vi "Calculate Spot Profile (SubVI).vi"(0 "step":sgl=0.1, 1 "z":sgl, 5 "N points":i32=16, 6 "CUDA/SLM error out":errorcluster, 7 "y":sgl, 8 "CGH out":u8[][](array[numeric]), 9 "x":sgl, 10 "xz-plane":bool) -> (2 "error out":errorcluster, 3 "Spot profile":sgl[][](graph)=[[0.054696757, 0.08603831, 0.118001305, 0.14888857, 0.17700168, 0.20075542, 0.21878594, 0.23004508, 0.2338732, 0.23004507, 0.21878591, 0.20075536, 0.17700155, 0.14888844, 0.118001245, 0.08603819], [0.086038314, 0.13533889, 0.18561684, 0.23420273, 0.27842486, 0.3157896, 0.34415174, 0.36186245, 0.36788404, 0.36186242, 0.34415168, 0.31578955, 0.27842474, 0.23420255, 0.18561675, 0.13533843], [0.118001334, 0.18561685, 0.25457302, 0.32120848, 0.38185897, 0.43310463, 0.47200322, 0.4962935, 0.50455207, 0.49629346, 0.4720032, 0.43310457, 0.3818589, 0.32120833, 0.25457323, 0.1856167], [0.14888862, 0.23420276, 0.3212085, 0.40528595, 0.48181203, 0.54647136, 0.5955519, 0.62620014, 0.63662064, 0.62620014, 0.5955518, 0.54647136, 0.48181185, 0.40528563, 0.32120845, 0.23420261], [0.17700171, 0.27842495, 0.38185903, 0.4818121, 0.5727876, 0.6496562, 0.708004, 0.74443936, 0.75682706, 0.74443924, 0.7080039, 0.649656, 0.5727872, 0.48181182, 0.38185894, 0.2784247], [0.20075557, 0.31578973, 0.43310472, 0.5464715, 0.64965636, 0.7368403, 0.80301875, 0.84434366, 0.8583939, 0.8443436, 0.8030185, 0.7368401, 0.6496561, 0.54647136, 0.43310463, 0.31578952], [0.21878609, 0.34415194, 0.47200343, 0.5955521, 0.7080042, 0.8030188, 0.87514055, 0.9201772, 0.93548924, 0.9201771, 0.87514055, 0.80301857, 0.708004, 0.59555185, 0.47200337, 0.3441517], [0.23004533, 0.36186272, 0.49629375, 0.62620044, 0.7444396, 0.8443437, 0.9201771, 0.9675313, 0.9836316, 0.9675312, 0.9201771, 0.84434366, 0.74443936, 0.62620026, 0.49629363, 0.36186248], [0.23387356, 0.36788428, 0.5045524, 0.6366208, 0.75682765, 0.8583941, 0.9354895, 0.9836317, 1.0, 0.9836316, 0.9354894, 0.85839397, 0.75682753, 0.6366205, 0.50455236, 0.36788407], [0.23004536, 0.36186272, 0.49629378, 0.62620044, 0.74443954, 0.8443438, 0.9201772, 0.9675312, 0.98363173, 0.9675312, 0.92017716, 0.84434366, 0.7444395, 0.62620014, 0.4962937, 0.36186248], [0.2187862, 0.34415203, 0.47200355, 0.59555215, 0.70800436, 0.8030188, 0.87514067, 0.9201771, 0.9354895, 0.9201772, 0.87514067, 0.8030187, 0.7080041, 0.59555197, 0.47200346, 0.34415174], [0.20075566, 0.3157898, 0.43310487, 0.54647166, 0.6496564, 0.7368404, 0.80301875, 0.8443438, 0.85839415, 0.8443437, 0.8030187, 0.7368404, 0.6496562, 0.5464714, 0.43310475, 0.3157896], [0.17700182, 0.27842504, 0.38185915, 0.48181218, 0.57278764, 0.64965636, 0.70800424, 0.74443954, 0.7568273, 0.7444395, 0.7080042, 0.64965624, 0.5727876, 0.481812, 0.38185906, 0.27842483], [0.14888875, 0.23420288, 0.3212086, 0.40528595, 0.48181215, 0.5464716, 0.5955521, 0.6262004, 0.63662094, 0.62620026, 0.595552, 0.5464714, 0.481812, 0.40528595, 0.32120848, 0.23420265], [0.11800147, 0.18561701, 0.2545734, 0.3212087, 0.38185927, 0.43310502, 0.4720036, 0.49629375, 0.5045525, 0.49629375, 0.47200346, 0.4331049, 0.3818591, 0.32120848, 0.25457317, 0.18561685], [0.0860384, 0.13533875, 0.18561698, 0.23420288, 0.27842504, 0.3157898, 0.34415194, 0.36186266, 0.36788437, 0.3618626, 0.34415185, 0.31578973, 0.2784249, 0.23420271, 0.18561687, 0.1353389]], 4 "return":i32)   [LabVIEW 2009]
uses:
  GenerateHologramCUDA.dll
panel:
  out "Computation Time":dbl
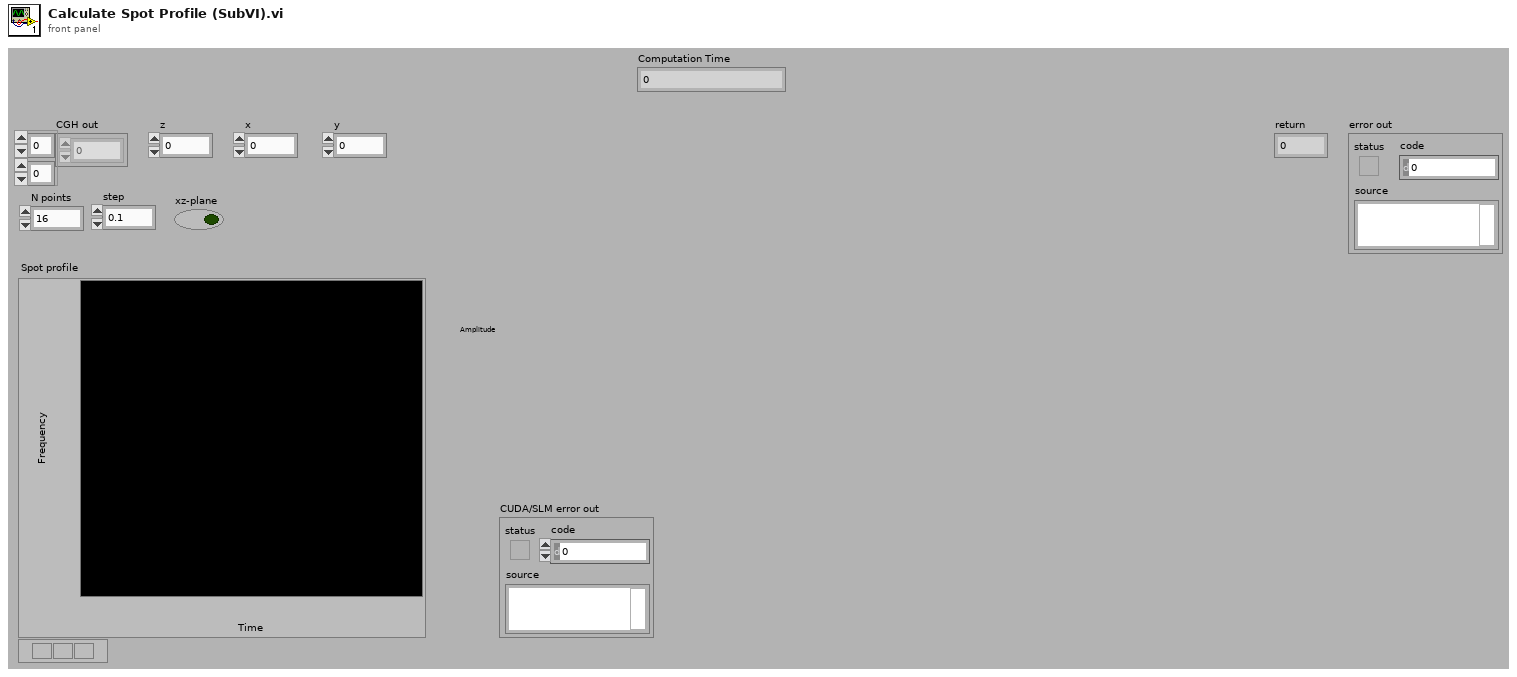
[diagram p1: front panel]
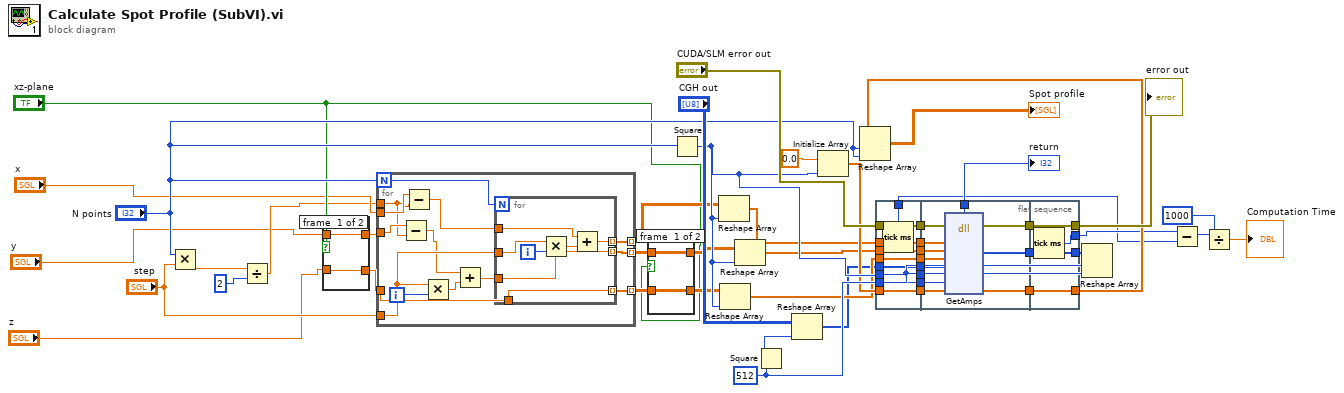
[diagram p0: block diagram]
diagram:
  w47 = 512 ("dimension size")
  n1 = Multiply(x="N points", y="step") -> (x*y=w31:sgl)
  n2 = Divide(x=w31, y=2) -> (x/y=w19:sgl)
  n3 = case shown="True" "xz-plane" {
    tunnel: "y" -> [w50 w51]
    tunnel: [w50 w52] -> w28
    tunnel: "z" -> [w49 w52]
    tunnel: [w49 w51] -> w26
    frame #0 {
    }
    frame #1 {
    }
  }
  n4 = for {
    N: "N points" -> [w58]
    tunnel: "step" -> [w64]
    tunnel: w28 -> [w55]
    tunnel: [w63] -> w34 mode=indexing
    tunnel: [w62] -> w25 mode=indexing
    tunnel: w26 -> [w61]
    tunnel: [w60] -> w23 mode=indexing
    tunnel: "x" -> [w57]
    tunnel: w19 -> [w53]
    i -> [w65]
    n5 = Subtract(x=w55, y=w53) -> (x-y=w54:sgl)
    n6 = Subtract(x=w57, y=w53) -> (x-y=w56:sgl)
    n7 = Multiply(x=w64, y=w65) -> (x*y=w66:sgl)
    n8 = Add(x=w54, y=w66) -> (x+y=w59:sgl)
    n9 = for {
      N: w58 -> [_]
      tunnel: w56 -> [w73]
      tunnel: w64 -> [w71]
      tunnel: [w69] -> w62 mode=indexing
      tunnel: w59 -> [w69]
      tunnel: [w68] -> w63 mode=indexing
      tunnel: w61 -> [w67]
      tunnel: [w67] -> w60 mode=indexing
      i -> [w72]
      n10 = Multiply(x=w71, y=w72) -> (x*y=w70:sgl)
      n11 = Add(x=w73, y=w70) -> (x+y=w68:sgl)
    }
  }
  n12 = case shown="True" "xz-plane" {
    tunnel: w25 -> [w75 w76]
    tunnel: [w75 w77] -> w24
    tunnel: w23 -> [w74 w77]
    tunnel: [w74 w76] -> w22
    frame #0 {
    }
    frame #1 {
    }
  }
  n13 = Square(x="N points") -> (x^2=w42:i32)
  n14 = Reshape Array(w34, w42) -> (w35:sgl[])
  n15 = Reshape Array(w22, w42) -> (w37:sgl[])
  n16 = Reshape Array(w24, w42) -> (w36:sgl[])
  n17 = Square(x=w47) -> (x^2=w29:i32)
  n18 = Reshape Array("CGH out", w29) -> (w30:u8[])
  n19 = Initialize Array(sgl 0.0 ("element"), w42) -> (w39:sgl[])
  n20 = Reshape Array(w40, "N points", "N points") -> (→"Spot profile":sgl[][])
  n21 = flat-sequence {
    tunnel: w30 -> [w79]
    tunnel: w35 -> [w80]
    tunnel: w36 -> [w81]
    tunnel: w37 -> [w82]
    tunnel: w39 -> [w83]
    tunnel: w42 -> [w84]
    tunnel: "CUDA/SLM error out" -> [w85]
    tunnel: w47 -> [w86]
    tunnel: [w86] -> w14
    tunnel: [w85] -> w13
    tunnel: [w84] -> w12
    tunnel: [w83] -> w11
    tunnel: [w82] -> w10
    tunnel: [w81] -> w9
    tunnel: [w80] -> w8
    tunnel: [w79] -> w7
    tunnel: [w78] -> w2
    tunnel: [w96] -> w45
    tunnel: [w97] -> w17
    tunnel: [w94] -> w16
    tunnel: [w92] -> w15
    tunnel: w14 -> [w98]
    tunnel: w13 -> [w95]
    tunnel: w12 -> [w93]
    tunnel: w11 -> [w91]
    tunnel: w10 -> [w90]
    tunnel: w9 -> [w89]
    tunnel: w8 -> [w88]
    tunnel: w7 -> [w87]
    tunnel: [w100] -> w40
    tunnel: [w101] -> w43
    tunnel: [w102] -> w46
    tunnel: w17 -> [w102]
    tunnel: w16 -> [w101]
    tunnel: w15 -> [w100]
    tunnel: [w99] -> w3
    frame #0 {
      n22 = Tick Count (ms)() -> (millisecond timer value=w78:u32)
    }
    frame #1 {
      n23 = dll-call lib="C:/Users/Martin/Dropbox/GU/CUDA/GenerateHologramCUDA/LabVIEW/GenerateHologramCUDA.dll" fn="GetAmps"(error in=w95, "x"=w88, "y"=w89, "z"=w90, "Hologram"=w87, "N_spots"=w93, "SLM_size"=w98, "spot_amps"=w91) -> (error out=w94:errorcluster, "return"=w96:i32, "Hologram"=w97:u8[], "spot_amps"=w92:sgl[])  [unwired: 7 in, 1 out]
    }
    frame #2 {
      n24 = Tick Count (ms)() -> (millisecond timer value=w99:u32)
    }
  }
  n25 = Reshape Array(w46, w47, w47) -> ()  [unwired: 1 out]
  n26 = Subtract(x=w3, y=w2) -> (x-y=w6:u32)
  n27 = Divide(x=w6, y=u32 1000) -> (x/y=→"Computation Time":dbl)
  "return" <- w45
  "error out" <- w43
